vi "SParam Close Session.vi"(8 "error in":errorcluster, 11 "S-Par Reference In":T1) -> (0 "error out":errorcluster)   [LabVIEW 2023]
uses:
  <vilib>/niSPML/Typedefs/Session Handle.ctl
  <vilib>/niSPML/S-Par Reference.lvclass
  <vilib>/niSPML/Get Topology References (2CperPort1VST).vi
  <vilib>/niSPML/S-Parameter Measurements.lvlib
  <vilib>/niSPML/Switching/2 Couplers Per Port 1 VST/S-Par 2 Couplers Per Port 1 VST Switching.lvclass
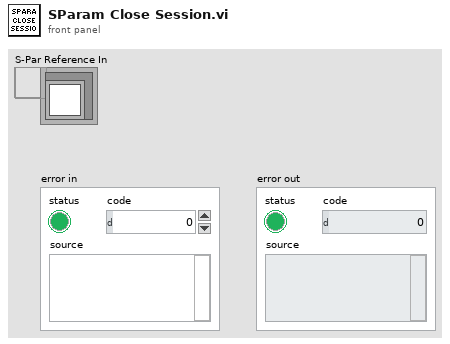
[diagram p1: front panel]
types:
  T1 = typedef "S-Parameter Measurements.lvlib/S-Par Reference.lvclass/Session Handle.ctl" = refnum<data-value>
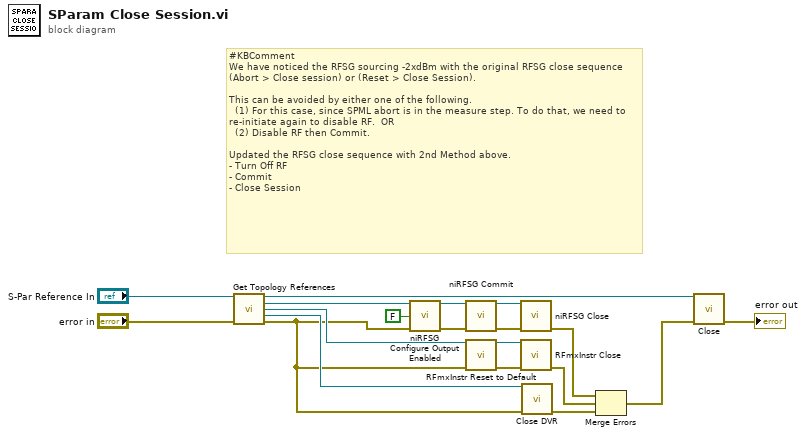
[diagram p0: block diagram]
diagram:
  # "#KBComment\nWe have noticed the RFSG sourcing -2xdBm with the original RFSG close sequence (Abort > Close session) or (Reset > Close Session). \n\nThis can be avoided by either one of the following. \n  (1) For this case, since SPML abort is in the measure step. To do that, we need to re-initiate again to disable RF.  OR\n  (2) Disable RF then Commit.\n\nUpdated the RFSG close sequence with 2nd Method above. \n- Turn Off RF\n- Commit\n- Close Session"
  n1 = call-poly <vilib>:"Get Topology References.vi"("S-Par Reference In"="S-Par Reference In", "error in"="error in") -> ("S-Par Reference Out"=w19:T1, "NI RFSG Session"=w6:refnum<k15>, "NI RFmx Session"=w10:refnum<k21>, "Switch Reference"=w14:refnum<data-value>, "error out"=w5:errorcluster)  [unwired: 9 in]
  n2 = call <instrlib>:"niRFSG Configure Output Enabled.vi"("instrument handle"=w6, "output enabled"=FALSE, "error in"=w5) -> ("instrument handle out"=w4:refnum<k15>, "error out"=w3:errorcluster)  [unwired: 11 in]
  n3 = call <instrlib>:"niRFSG Commit.vi"("instrument handle"=w4, "error in"=w3) -> ("instrument handle out"=w2:refnum<k15>, "error out"=w1:errorcluster)  [unwired: 12 in]
  n4 = call <vilib>:"RFmxInstr Reset to Default.vi"("Instrument Handle In"=w10, "error in (no error)"=w5) -> ("Instrument Handle Out"=w9:refnum<k21>, "error out"=w8:errorcluster)  [unwired: 12 in]
  n5 = call <instrlib>:"niRFSG Close.vi"("instrument handle"=w2, "error in"=w1) -> ("error out"=w17:errorcluster)  [unwired: 13 in]
  n6 = call <vilib>:"RFmxInstr Close.vi"("Instrument Handle In"=w9, "error in (no error)"=w8) -> ("error out"=w16:errorcluster)  [unwired: 13 in]
  n7 = call <vilib>:"Close DVR.vi"("error in (no error)"=w5, "Switching Reference"=w14) -> ("error out"=w15:errorcluster)  [unwired: 9 in]
  n8 = Merge Errors(w17, w16, w15) -> (w18:errorcluster)
  n9 = call <vilib>:"Close.vi"("S-Par Reference In"=w19, "error in"=w18) -> ("error out"=→"error out":errorcluster)  [unwired: 13 in]
